vi "Set Parallel Test Return Data.vi"(8 "error in (no error)":errorcluster, 10 "Parallel Test Return Data":T1, 11 "Parallel Test in":refnum<class "Parallel Test.lvclass">) -> (0 "error out":errorcluster, 3 "Parallel Test out":refnum<class "Parallel Test.lvclass">)   [LabVIEW 2015, in "Parallel Test.lvclass"]
uses:
  Parallel Test.lvclass
  typedefs/Parallel Return -- Cluster.ctl
  Parallel Test.lvclass/Parallel Test.ctl
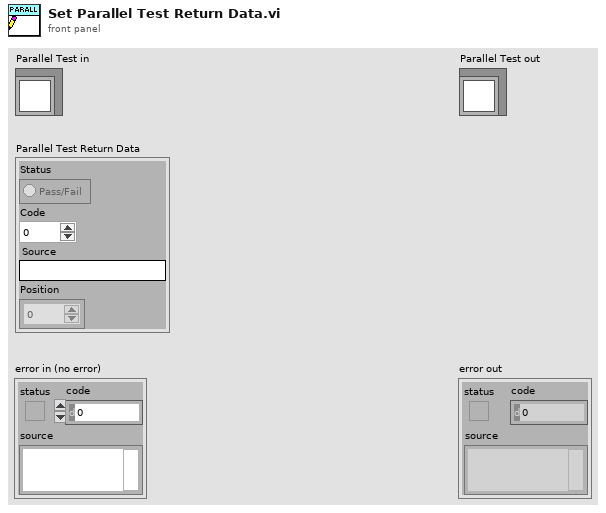
[diagram p1: front panel]
types:
  T1 = typedef "Parallel Test.lvclass/Parallel Return -- Cluster.ctl" = cluster{"Status":bool[], "Code":i32, "Source":string, "Position":u32[]}
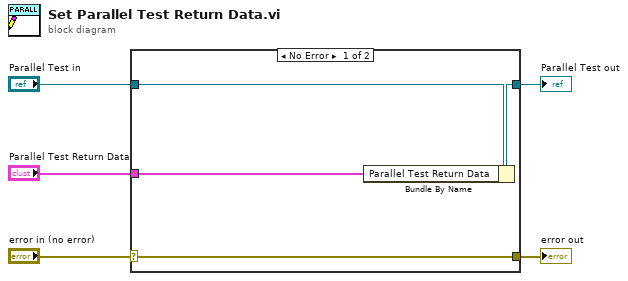
[diagram p0: block diagram]
diagram:
  n1 = case shown="No Error" "error in (no error)" {
    selector: "error in (no error)" -> [w9 w10]
    tunnel: [w9 w10] -> w4
    tunnel: [w7 w11] -> w2
    tunnel: "Parallel Test in" -> [w8 w11]
    tunnel: "Parallel Test Return Data" -> [w6 _]
    frame No Error {
      n2 = Bundle By Name(cluster=w8, "Parallel Test Return Data"=w6) -> (w7:refnum<class "Parallel Test.lvclass">)
    }
    frame Error {
    }
  }
  "error out" <- w4
  "Parallel Test out" <- w2
